vi "3-5-3.vi"() -> ()   [LabVIEW 2016]
uses:
  <vilib>/Utility/miscctls.llb/LVPoint32TypeDef.ctl
panel:
  out "new picture":picture
  in  "input image":path
  out "Vertical":i32(knob) scale=0.0..1000.0
  out "Horizontal":i32(knob) scale=0.0..1000.0
  in  "stop":bool
  out "Coords":T1
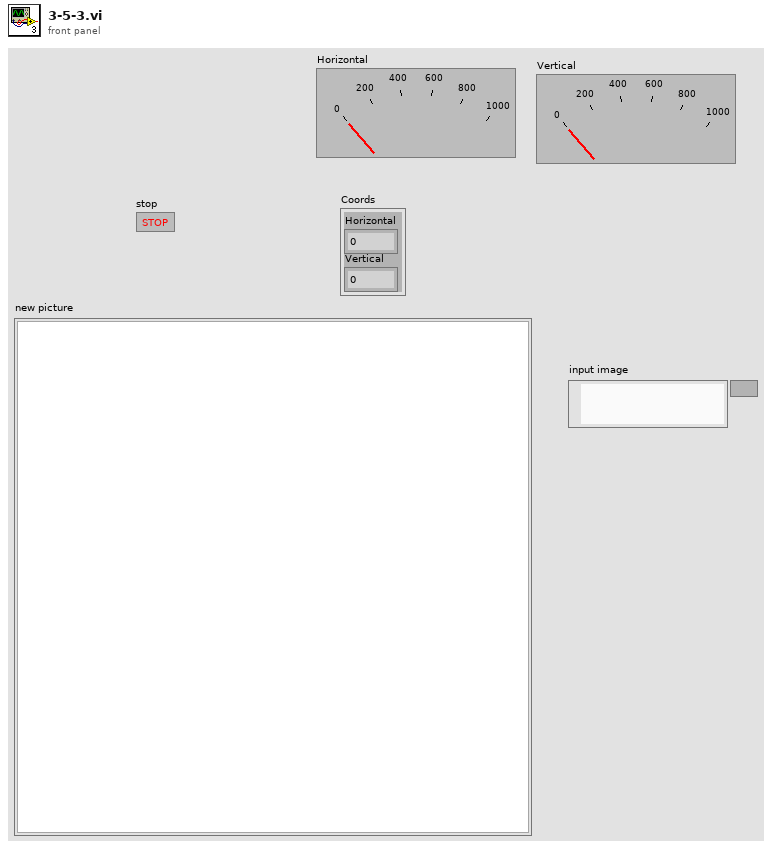
[diagram p1: front panel]
types:
  T1 = typedef "LVPoint32TypeDef.ctl" = cluster{"Horizontal":i32, "Vertical":i32}
  T2 = typedef "imagedata.ctl" = cluster{"image type":i32, "image depth":i32, "image":u8[], "mask":u8[], "colors":u32[], "Rectangle":cluster{"left":i16, "top":i16, "right":i16, "bottom":i16}}
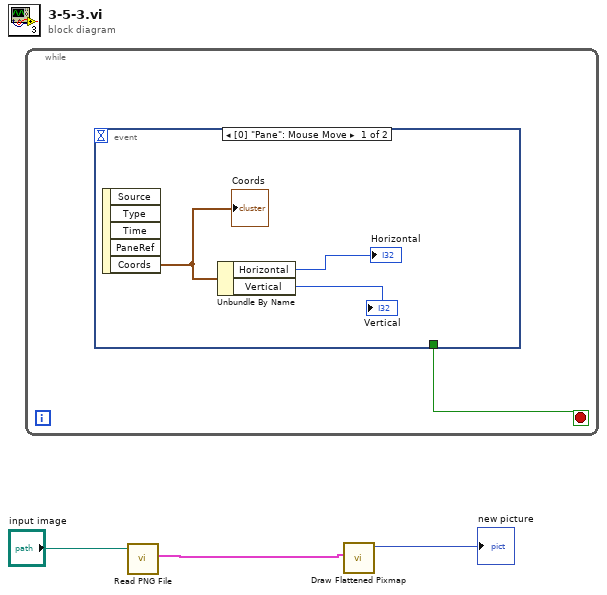
[diagram p0: block diagram]
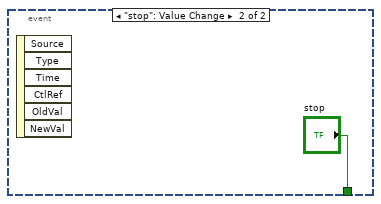
[diagram p2: hidden frame]
diagram:
  n1 = while {
    stop <- w4 stop-if-true
    n2 = event shown="[0] \"Pane\": Mouse Move" {
      selector: _ -> [_ _]
      dyn-events: _ -> [_ _]
      timeout: _ -> [_ _]
      tunnel: [_ "stop"] -> w4
      event Mouse Move {
        n3 = event-data() -> ("Coords"=w7:T1)  [unwired: 1 in, 4 out]
        "Coords" <- w7
        n4 = Unbundle By Name(w7) -> ("Horizontal"=→"Horizontal":i32, "Vertical"=→"Vertical":i32)
      }
      event "stop": Value Change {
        n5 = event-data() -> ()  [unwired: 1 in, 6 out]
      }
    }
  }
  n6 = call <vilib>:"Read PNG File.vi"("path to PNG file"="input image") -> ("image data"=w1:T2)  [unwired: 8 in, 2 out]
  n7 = call <vilib>:"Draw Flattened Pixmap.vi"("image data"=w1) -> ("new picture"=→"new picture":picture)  [unwired: 8 in]
